vi "_시리얼-패킷 데이타-수신 - GEN4 1st PP - 전체처리.vi"(5 "CDC Offet":T1 caption="CDC Offset data" {"Right Wing-C, C6/C0" format="%#.9f"; "Right Wing-B, C5/C0" format="%#.9f"; "Right Wing-A, C4/C0" format="%#.9f"; "Left Wing-C, C3/C0" format="%#.9f"; "Left Wing-B, C2/C0" format="%#.9f"; "Left Wing-A, C1/C0" format="%#.9f"}, 6 "필터 적용":bool, 7 "시리얼 포트":refnum<visa-resource-name>="COM9") -> (1 "CDC data":T1 caption="CDC Monitoring data" {"Right Wing-C, C6/C0" format="%#.9f"; "Right Wing-B, C5/C0" format="%#.9f"; "Right Wing-A, C4/C0" format="%#.9f"; "Left Wing-C, C3/C0" format="%#.9f"; "Left Wing-B, C2/C0" format="%#.9f"; "Left Wing-A, C1/C0" format="%#.9f"}, 2 "*Board ID1":string="None...." caption="F/W Ver.", 3 "수신 실패(T)":bool)   [LabVIEW 2015]
panel:
  # "CDC 수신 데이터 처리/변환"
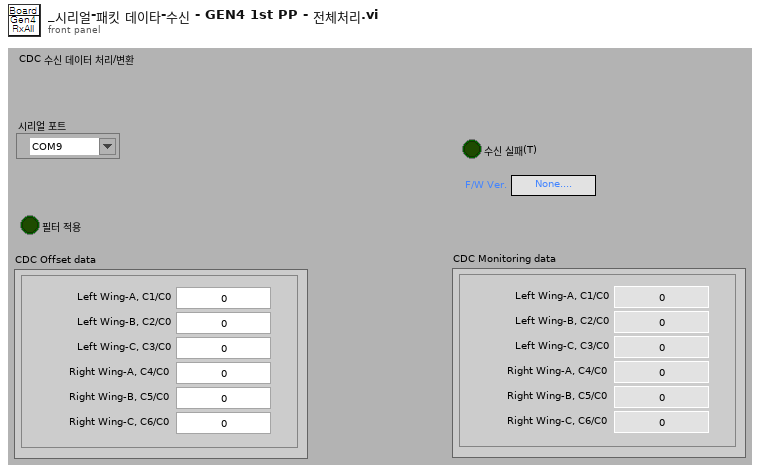
[diagram p1: front panel]
types:
  T1 = typedef "컨트롤-CDC data.ctl" = cluster{"Left Wing-A, C1/C0":dbl, "Left Wing-B, C2/C0":dbl, "Left Wing-C, C3/C0":dbl, "Right Wing-A, C4/C0":dbl, "Right Wing-B, C5/C0":dbl, "Right Wing-C, C6/C0":dbl}
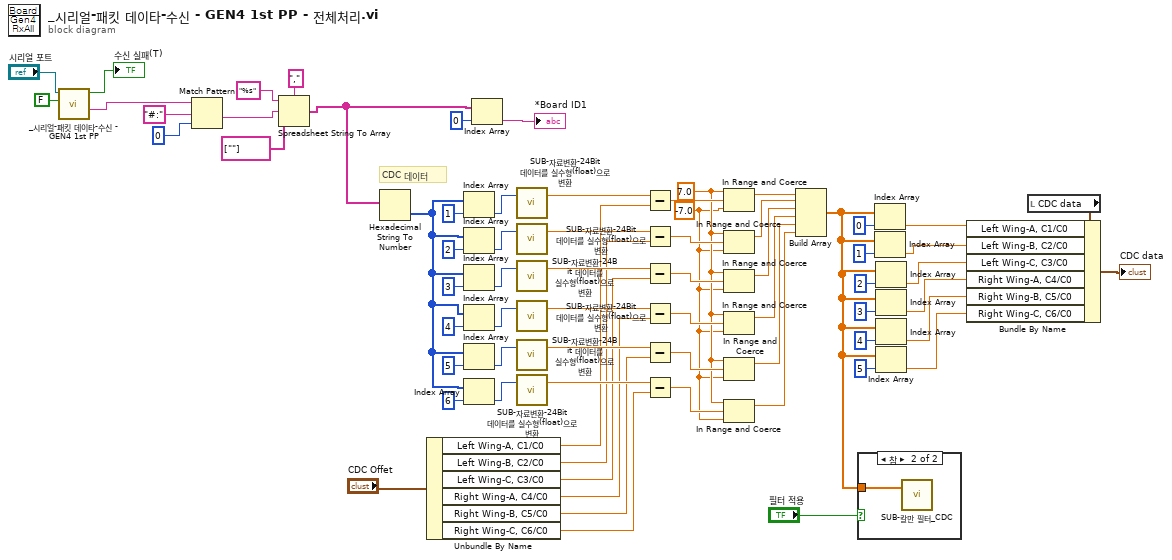
[diagram p0: block diagram]
diagram:
  w34 = 7.0 ("상위 리미트")
  w33 = -7.0 ("하위 리미트")
  # "CDC 데이터"
  n1 = call "_시리얼-패킷 데이타-수신 - GEN4 1st PP.vi"("ErrIn"=FALSE, "시리얼 포트"="시리얼 포트") -> ("수신 문자열"=w61:string, "수신 실패(T)"=→"수신 실패(T)":bool)  [unwired: 2 in, 2 out]
  n2 = Match Pattern(string=w61, regular expression="#:" ("검색 문자열"), offset (0)=0 ("오프셋(0)")) -> (after substring=w62:string)  [unwired: 3 out]
  n3 = Spreadsheet String To Array(delimiter (Tab)="," ("구분 문자(탭)"), format string="%s" ("스프레드시트 문자열"), spreadsheet string=w62, array type (2D Dbl)=string[] [""] ("배열 타입(2D Dbl)")) -> (array=w12:string[])
  n4 = Hexadecimal String To Number(string=w12) -> (number=w14:u32[])  [unwired: 2 in, 1 out]
  n5 = Unbundle By Name("CDC Offet") -> ("Left Wing-A, C1/C0"=w6:dbl, "Left Wing-B, C2/C0"=w5:dbl, "Left Wing-C, C3/C0"=w4:dbl, "Right Wing-A, C4/C0"=w3:dbl, "Right Wing-B, C5/C0"=w2:dbl, "Right Wing-C, C6/C0"=w1:dbl)
  n6 = Index Array(array=w14, index=1 ("인덱스")) -> (element=w57:u32)
  n7 = Index Array(array=w14, index=2 ("인덱스")) -> (element=w52:u32)
  n8 = Index Array(array=w14, index=3 ("인덱스")) -> (element=w44:u32)
  n9 = Index Array(array=w14, index=4 ("인덱스")) -> (element=w49:u32)
  n10 = Index Array(array=w14, index=5 ("인덱스")) -> (element=w41:u32)
  n11 = Index Array(array=w14, index=6 ("인덱스")) -> (element=w36:u32)
  n12 = Index Array(array=w12, index=0 ("인덱스")) -> (element=→"*Board ID1":string)
  n13 = call "SUB-자료변환-24Bit 데이터를 실수형(float)으로 변환.vi"("U32"=w57) -> ("FP32"=w56:sgl)  [unwired: 2 in]
  n14 = call "SUB-자료변환-24Bit 데이터를 실수형(float)으로 변환.vi"("U32"=w52) -> ("FP32"=w53:sgl)  [unwired: 2 in]
  n15 = call "SUB-자료변환-24Bit 데이터를 실수형(float)으로 변환.vi"("U32"=w44) -> ("FP32"=w45:sgl)  [unwired: 2 in]
  n16 = call "SUB-자료변환-24Bit 데이터를 실수형(float)으로 변환.vi"("U32"=w49) -> ("FP32"=w48:sgl)  [unwired: 2 in]
  n17 = call "SUB-자료변환-24Bit 데이터를 실수형(float)으로 변환.vi"("U32"=w41) -> ("FP32"=w40:sgl)  [unwired: 2 in]
  n18 = call "SUB-자료변환-24Bit 데이터를 실수형(float)으로 변환.vi"("U32"=w36) -> ("FP32"=w37:sgl)  [unwired: 2 in]
  n19 = Subtract(x=w56, y=w6) -> (x-y=w55:dbl)
  n20 = Subtract(x=w53, y=w5) -> (x-y=w54:dbl)
  n21 = Subtract(x=w45, y=w4) -> (x-y=w46:dbl)
  n22 = Subtract(x=w48, y=w3) -> (x-y=w47:dbl)
  n23 = Subtract(x=w40, y=w2) -> (x-y=w39:dbl)
  n24 = Subtract(x=w37, y=w1) -> (x-y=w38:dbl)
  n25 = In Range and Coerce(upper limit=w34, x=w55, lower limit=w33) -> (coerced(x)=w15:dbl)  [unwired: 1 out]
  n26 = In Range and Coerce(upper limit=w34, x=w54, lower limit=w33) -> (coerced(x)=w32:dbl)  [unwired: 1 out]
  n27 = In Range and Coerce(upper limit=w34, x=w46, lower limit=w33) -> (coerced(x)=w31:dbl)  [unwired: 1 out]
  n28 = In Range and Coerce(upper limit=w34, x=w47, lower limit=w33) -> (coerced(x)=w30:dbl)  [unwired: 1 out]
  n29 = In Range and Coerce(upper limit=w34, x=w39, lower limit=w33) -> (coerced(x)=w29:dbl)  [unwired: 1 out]
  n30 = In Range and Coerce(upper limit=w34, x=w38, lower limit=w33) -> (coerced(x)=w13:dbl)  [unwired: 1 out]
  n31 = Build Array(w15, w32, w31, w30, w29, w13) -> (w9:dbl[])
  n32 = case shown="참" "필터 적용" {
    tunnel: w9 -> [_ w70]
    frame False {
    }
    frame True {
      n33 = call "SUB-칼만 필터_CDC.vi"("x set"=w70) -> ()  [unwired: 2 in, 1 out]
    }
  }
  n34 = Index Array(array=w9, index=0 ("인덱스")) -> (element=w27:dbl)
  n35 = Index Array(array=w9, index=1 ("인덱스")) -> (element=w26:dbl)
  n36 = Index Array(array=w9, index=2 ("인덱스")) -> (element=w25:dbl)
  n37 = Index Array(array=w9, index=3 ("인덱스")) -> (element=w24:dbl)
  n38 = Index Array(array=w9, index=4 ("인덱스")) -> (element=w23:dbl)
  n39 = Index Array(array=w9, index=5 ("인덱스")) -> (element=w22:dbl)
  n40 = local read "CDC data"() -> (w28:T1)
  n41 = Bundle By Name(cluster=w28, "Left Wing-A, C1/C0"=w27, "Left Wing-B, C2/C0"=w26, "Left Wing-C, C3/C0"=w25, "Right Wing-A, C4/C0"=w24, "Right Wing-B, C5/C0"=w23, "Right Wing-C, C6/C0"=w22) -> (→"CDC data":T1)
